vi "Update Values with Terminals Status.vi"(8 "error in":errorcluster, 10 "values in":dbl[](array[numeric]), 11 "Rx execution unit in":refnum<class "Rx Execution Unit.lvclass">) -> (0 "error out":errorcluster, 2 "values out":dbl[](array[numeric]), 3 "Rx execution unit out":refnum<class "Rx Execution Unit.lvclass">)   [LabVIEW 2020, in "Ballard MIL-STD-1553 Engine.lvlib" / "Implementation.lvlib" / "Rx Execution Unit.lvclass"]
uses:
  Rx Execution Unit.lvclass
  Rx Execution Unit.lvclass/Rx Execution Unit.ctl
  <instrlib>/BTI1553Lib/BTI1553LV.lvlib
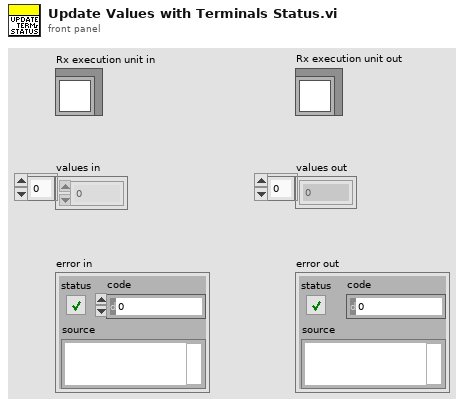
[diagram p1: front panel]
types:
  T1 = typedef "Ballard MIL-STD-1553 Engine.lvlib/Implementation.lvlib/Rx Execution Unit.lvclass/Status Terminal Lookup Data.ctl" = cluster{"value index":i32, "remote terminal handle":u64, "terminal address":u64}
  T2 = typedef "BTI1553LV.lvlib/1553 BC Status.ctl" = u32
  T3 = typedef "BTI1553LV.lvlib/1553 RT Status.ctl" = u32
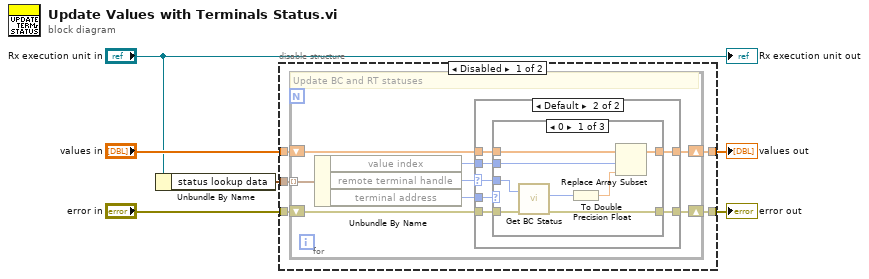
[diagram p0: block diagram]
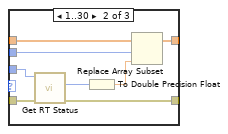
[diagram p3: hidden frame]
diagram:
  n1 = Unbundle By Name("Rx execution unit in") -> ("status lookup data"=w3:T1[])
  n2 = disable-structure shown="Disabled" {
    disable-tunnel: [w11 w47] -> w6
    disable-tunnel: [w10 w48] -> w5
    disable-tunnel: "error in" -> [w9 w48]
    disable-tunnel: w3 -> [w8 _]
    disable-tunnel: "values in" -> [w7 w47]
    frame Disabled {
      n3 = for {
        tunnel: w8 -> [w18] mode=indexing
        shift-right: [w16] -> w10
        shift-left: w9 -> [w17]
        shift-right: [w12] -> w11
        shift-left: w7 -> [w13]
        # "Update BC and RT statuses"
        n4 = Unbundle By Name(w18) -> ("value index"=w14:i32, "remote terminal handle"=w19:u64, "terminal address"=w15:u64)
        n5 = case shown="Default" w19 {
          selector: w19 -> [_ w28]
          tunnel: w17 -> [w20 w27]
          tunnel: [w20 w26] -> w16
          tunnel: w15 -> [_ w25]
          tunnel: w14 -> [_ w24]
          tunnel: w13 -> [w21 w23]
          tunnel: [w21 w22] -> w12
          frame 0, -1 {
          }
          frame Default {
            n6 = case shown="0" w25 {
              tunnel: w27 -> [w35 w43 w46]
              tunnel: w28 -> [w36 w44 _]
              tunnel: [w34 w42 w46] -> w26
              tunnel: w24 -> [w32 w40 _]
              tunnel: w23 -> [w30 w38 w45]
              tunnel: [w29 w37 w45] -> w22
              frame 0 {
                # "RTs"
                n7 = call <instrlib>:"Get BC Status.vi"("error in (no error)"=w35, "bus controller handle in"=w36) -> ("error out"=w34:errorcluster, "status"=w31:T2)  [unwired: 7 in, 1 out]
                n8 = To Double Precision Float(number=w31) -> (double precision float=w33:dbl)
                n9 = Replace Array Subset(array=w30, new element=w33, index=w32) -> (w29:dbl[])
              }
              frame 1..30 {
                # "RTs"
                n10 = call <instrlib>:"Get RT Status.vi"("error in (no error)"=w43, "remote terminal handle in"=w44) -> ("error out"=w42:errorcluster, "status"=w39:T3)  [unwired: 7 in, 1 out]
                n11 = To Double Precision Float(number=w39) -> (double precision float=w41:dbl)
                n12 = Replace Array Subset(array=w38, new element=w41, index=w40) -> (w37:dbl[])
              }
              frame Default {
                # "BC"
              }
            }
          }
        }
      }
    }
    frame Enabled {
    }
  }
  "values out" <- w6
  "error out" <- w5
  "Rx execution unit out" <- "Rx execution unit in"
